vi "Stop Core.vi"(10 "final error code":i32, 11 "Test Node Charm View in":refnum<class "Test Node Charm View.lvclass">) -> (3 "Test Node Charm View out":refnum<class "Test Node Charm View.lvclass">)   [LabVIEW 2013, in "Test Node Charm View.lvlib" / "Test Node Charm View.lvclass"]
doc: "(<B>Filename</B>: Actor Framework.lvlib:Actor.lvclass:Stop Core.vi)\n\nDefines what the actor does before it stops. Use the <B>final error code</B> input to determine whether the actor shut down in response to an error.\n\nBy default, this method does nothing. A descendant class may override it to define behavior, such as shutting down any processes the actor initiated in its override of the Actor Core method."
uses:
  Test Node Charm View.lvclass
  <vilib>/ActorFrameworkMVC/View Actor/View Actor.lvclass
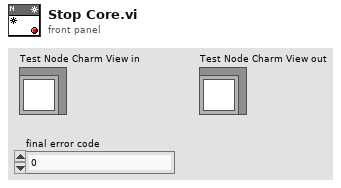
[diagram p1: front panel]
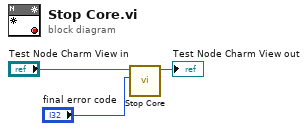
[diagram p0: block diagram]
diagram:
  n1 = call-parent "Stop Core.vi"("final error code"="final error code", "Actor in"="Test Node Charm View in") -> ("Actor out"=→"Test Node Charm View out":refnum<class "Test Node Charm View.lvclass">)  [unwired: 9 in]
